vi "niFPGA BFGroup Twiddle Table 512 U64.vi"(7 "address":fxp<+,9,9>) -> (4 "twid real":fxp<+/-,33,2> format="%.32g", 6 "twid imag":fxp<+/-,33,2> format="%.32g")   [LabVIEW 2017]
uses:
  <vilib>/Utility/error.llb/Clear Errors.vi
  <vilib>/rvi/Emulation/niFpgaSctlEmulationGetInTimedLoop.vi
  <vilib>/rvi/DataTransferAndStorage/Container/Common/niFpgaContainerGetUniqueNameForEmu.vi
  <vilib>/rvi/DataTransferAndStorage/Container/Common/niFpgaContainerSetEmuInfo.vi
  <vilib>/rvi/eio/common/nirviEmuReportErrorAndStop.vi
  <vilib>/rvi/Memory/Memory_Emulation/nirvimemoryEmulation.vi
  <vilib>/rvi/Memory/Memory_Emulation/nirvimemoryFastEmulation.vi
  <vilib>/rvi/Memory/Memory_Emulation/niFpgaMemoryEmulationCacheClearOnFirstRun.vi
  <vilib>/rvi/Memory/Memory_Emulation/nirvimemoryEmulationManagerCache_MakeExclusive.vi
  <vilib>/rvi/Memory/Memory_Emulation/niFpgaMemoryEmulationValidateCache.vi
  <vilib>/rvi/Memory/Memory_Emulation/nirvimemoryEmulationManagerCache_InsertValue.vi
  <vilib>/rvi/Memory/Memory_Emulation/nirvimemoryEmulationManagerCache_ReleaseExclusive.vi
  <vilib>/rvi/Memory/Memory_Emulation/nirvimemoryEmulationManagerCache_GetValue.vi
  <vilib>/rvi/Emulation/niFpgaEmulationIsFPGAContextNoSignature.vi
  <vilib>/rvi/Memory/Memory_Emulation/nirvimemoryEmulationManagerCache_SetValue.vi
  <vilib>/rvi/Emulation/niFpgaSctlEmulationResourceMgr.vi
  <vilib>/rvi/LocalResourceManager/LocalResourceManager.xnode
  <vilib>/rvi/DataTransferAndStorage/Container/XNode/niFpgaContainer.xnode
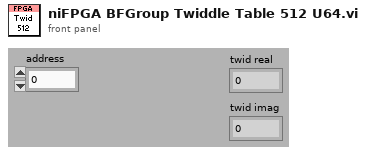
[diagram p1: front panel]
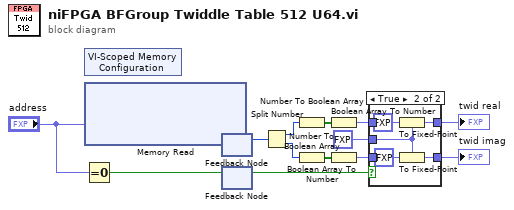
[diagram p0: block diagram]
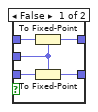
[diagram p2: hidden frame]
diagram:
  n1 = Equal To 0?(x="address") -> (x = 0?=w8:bool)
  n2 = xnode "VI-Scoped Memory Configuration"() -> ()  [unwired: 1 out]
  n3 = xnode ("Memory Read")("Address"="address") -> ("Data"=w14:u64)  [unwired: 2 out]
  n4 = feedback-in #1(w14) -> ()
  n5 = feedback #1() -> (w9:u64)  [unwired: 1 out]
  n6 = feedback-in #2(w8) -> ()
  n7 = feedback #2() -> (w1:bool)  [unwired: 1 out]
  n8 = Split Number(x=w9) -> (hi(x)=w12:u32, lo(x)=w10:u32)
  n9 = Number To Boolean Array(number=w12) -> (Boolean array=w13:bool[])
  n10 = Number To Boolean Array(number=w10) -> (Boolean array=w11:bool[])
  n11 = Boolean Array To Number(Boolean array=w13) -> (number=w5:fxp<+/-,32,1>)
  n12 = Boolean Array To Number(Boolean array=w11) -> (number=w3:fxp<+/-,32,1>)
  n13 = case shown="True" w1 {
    tunnel: w5 -> [w19 _]
    tunnel: [w18 w23] -> w4
    tunnel: w3 -> [w17 _]
    tunnel: [w16 w22] -> w2
    tunnel: fxp<+/-,33,2> 0.0 ("fixed-point type") -> [w15 w20]
    frame False {
      n14 = To Fixed-Point(fixed-point type=w15, number=w19) -> (fixed-point=w18:fxp<+/-,33,2>)
      n15 = To Fixed-Point(fixed-point type=w15, number=w17) -> (fixed-point=w16:fxp<+/-,33,2>)
    }
    frame True {
      n16 = To Fixed-Point(fixed-point type=w20, number=fxp<+,1,1> 1.0 ("fixed-point type")) -> (fixed-point=w23:fxp<+/-,33,2>)
      n17 = To Fixed-Point(fixed-point type=w20, number=fxp<+,1,1> 0.0 ("fixed-point type")) -> (fixed-point=w22:fxp<+/-,33,2>)
    }
  }
  "twid real" <- w4
  "twid imag" <- w2
